vi "sensitivity mso Measurement.vi"(0 "OSC":refnum<visa-resource-name>, 2 "Sensor Threshold Setting":dbl=1.005, 5 "Pace Voltage":dbl=1.5 format="%#_13g", 7 "Waveform Generator":refnum<visa-resource-name>, 9 "Delay":u32=8000, 11 "error in (no error)":errorcluster, 12 "Pace interval":dbl) -> (6 "Raw Data with OSC":waveform(dbl)[](array[waveform]), 10 "CH1 Waveform":waveform(dbl)(graph), 14 "Sensor Threshold":dbl, 15 "CH3 Waveform":waveform(dbl)(graph))   [LabVIEW 2016]
uses:
  <instrlib>/Agilent 6000 Series/Agilent 6000 Series.lvlib
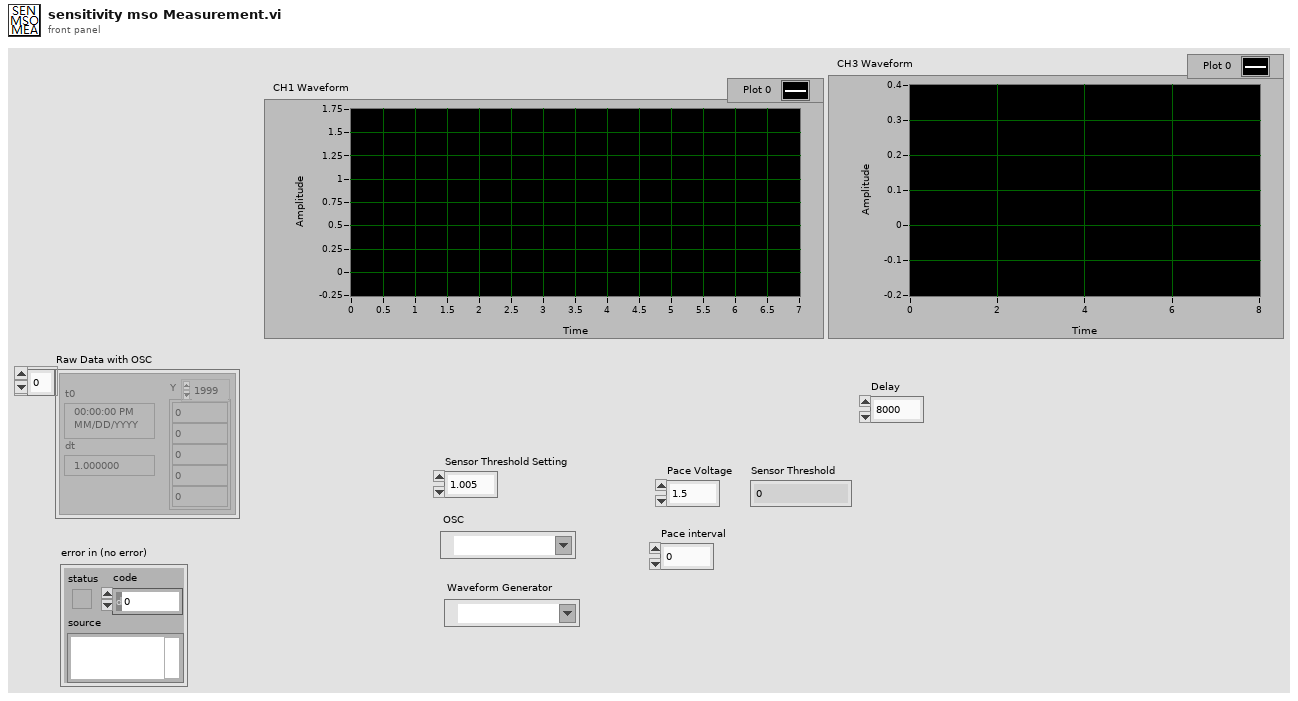
[diagram p1: front panel]
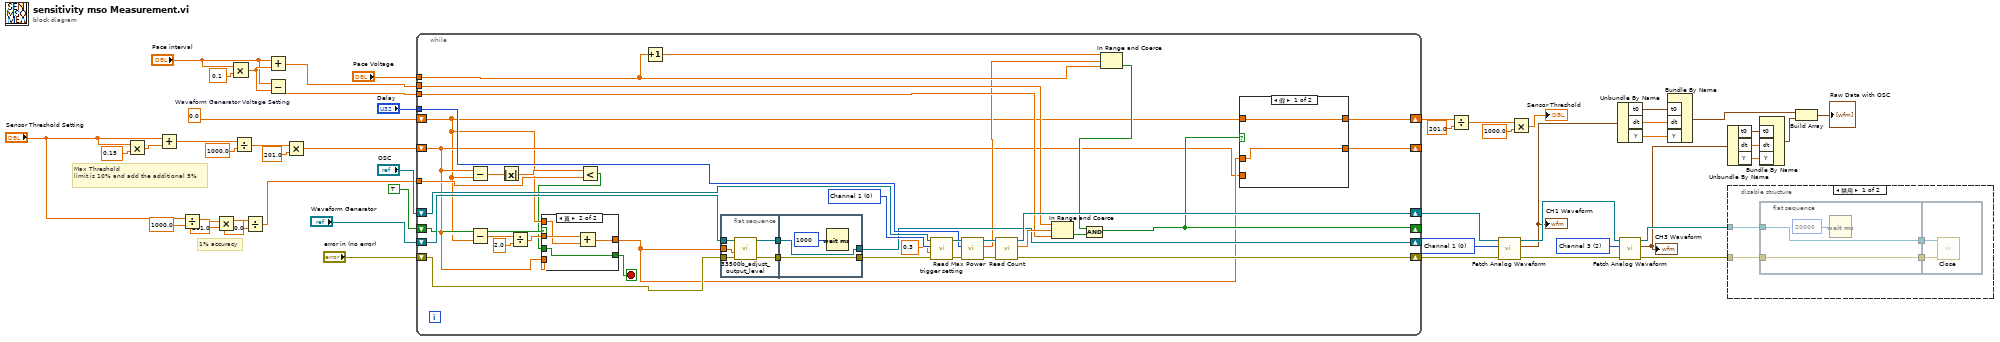
[diagram p0: block diagram]
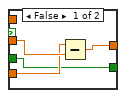
[diagram p2: hidden frame]
diagram:
  w9 = 0.0  # Waveform Generator Voltage Setting
  w48 = u16 2 items=["Channel 1", "Channel 2", "Channel 3", "Channel 4", "Math"] ("Source (0: Channel 1)")
  w50 = u16 0 items=["Channel 1", "Channel 2", "Channel 3", "Channel 4", "Math"] ("Source (0: Channel 1)")
  # "Max Threshold\nlimit is 10% and add the additional 5%"
  # "1% accuracy"
  n1 = Multiply(x="Sensor Threshold Setting", y=0.15) -> (x*y=w10:dbl)
  n2 = Add(x="Sensor Threshold Setting", y=w10) -> (x+y=w19:dbl)
  n3 = Divide(x="Sensor Threshold Setting", y=1000.0) -> (x/y=w5:dbl)
  n4 = Multiply(x=w5, y=201.0) -> (x*y=w3:dbl)
  n5 = Multiply(x="Pace interval", y=0.1) -> (x*y=w15:dbl)
  n6 = Divide(x=w19, y=1000.0) -> (x/y=w17:dbl)
  n7 = Divide(x=w3, y=100.0) -> (x/y=w1:dbl)
  n8 = Add(x="Pace interval", y=w15) -> (x+y=w13:dbl)
  n9 = Subtract(x="Pace interval", y=w15) -> (x-y=w14:dbl)
  n10 = Multiply(x=w17, y=201.0) -> (x*y=w23:dbl)
  n11 = while {
    shift-right: [w76] -> w31
    shift-left: "OSC" -> [w89]
    shift-right: [w77] -> w30
    shift-left: "error in (no error)" -> [w65]
    tunnel: "Delay" -> [w85]
    tunnel: "Pace Voltage" -> [w63]
    shift-right: [w59] -> w26
    shift-left: w9 -> [w53]
    shift-right: [w70] -> _
    shift-left: "Waveform Generator" -> [w71]
    shift-right: [w56] -> _
    shift-left: w23 -> [w54]
    tunnel: w14 -> [w73]
    tunnel: w13 -> [w72]
    shift-right: [w60] -> _
    shift-left: TRUE -> [w55]
    tunnel: w1 -> [w66]
    stop <- w51 stop-if-true
    w88 = u16 0 items=["Channel 1", "Channel 2", "Channel 3", "Channel 4", "DIG 0", "DIG 1", "DIG 2", "DIG 3", "DIG 4", "DIG 5", "DIG 6", "DIG 7", "DIG 8", "DIG 9", "DIG 10", "DIG 11", "DIG 12", "DIG 13", "DIG 14", "DIG 15", "Line", "External"] ("Trigger Source (0: Channel 1)")
    n12 = Subtract(x=w54, y=w53) -> (x-y=w81:dbl)
    n13 = Subtract(x=w54, y=w53) -> (x-y=w84:dbl)
    n14 = Absolute Value(x=w81) -> (abs(x)=w80:dbl)
    n15 = Divide(x=w84, y=2.0) -> (x/y=w58:dbl)
    n16 = Less?(x=w80, y=w66) -> (x < y?=w52:bool)
    n17 = case shown="真" w55 {
      tunnel: w58 -> [w92 w97]
      tunnel: [w93 w96] -> w57
      tunnel: w54 -> [w91 _]
      tunnel: w53 -> [_ w95]
      tunnel: w52 -> [w90 w94]
      tunnel: [w90 w94] -> w51
      frame False {
        n18 = Subtract(x=w91, y=w92) -> (x-y=w93:dbl)
      }
      frame True {
        n19 = Add(x=w97, y=w95) -> (x+y=w96:dbl)
      }
    }
    n20 = Increment(x=w63) -> (x+1=w64:dbl)
    n21 = flat-sequence {
      tunnel: w71 -> [w106]
      tunnel: w65 -> [w104]
      tunnel: [w105] -> w69
      tunnel: [w103] -> w68
      tunnel: w57 -> [w102]
      tunnel: [w109] -> w70
      tunnel: w69 -> [w109]
      tunnel: w68 -> [w107]
      tunnel: [w107] -> w67
      frame #0 {
        n22 = call "33500b_adjust_output_level.vi"("错误输入（无错误）"=w104, "Amp(vpp)"=w102, "Waveform Generator"=w106) -> ("错误输出"=w103:errorcluster, "Waveform Generator"=w105:refnum<visa-resource-name>)  [unwired: 7 in]
      }
      frame #1 {
        n23 = Wait (ms)(milliseconds to wait=u32 1000 ("等待时间（毫秒）")) -> ()  [unwired: 1 out]
      }
    }
    n24 = call "trigger setting.vi"("error in (no error)"=w67, "Trigger Level (0.0 V)"=0.3, "Trigger Source (0: Channel 1)"=w88, "OSC"=w89) -> ("error out"=w86:errorcluster, "OSC"=w87:refnum<visa-resource-name>)  [unwired: 6 in]
    n25 = call "Read Max Power.vi"("错误输入（无错误）"=w86, "Delay"=w85, "OSC Input"=w87) -> ("错误输出"=w78:errorcluster, "Pace Max Amp"=w62:dbl, "OSC Output"=w79:refnum<visa-resource-name>)  [unwired: 6 in]
    n26 = call "Read Count.vi"("错误输入（无错误）"=w78, "OSC Input"=w79) -> ("错误输出"=w77:errorcluster, "Pace Interval"=w75:dbl, "OSC Output"=w76:refnum<visa-resource-name>)  [unwired: 7 in]
    n27 = In Range and Coerce(upper limit=w72, x=w75, lower limit=w73) -> (In Range?=w74:bool)  [unwired: 1 out]
    n28 = In Range and Coerce(upper limit=w64, x=w62, lower limit=w63) -> (In Range?=w61:bool)  [unwired: 1 out]
    n29 = Compound Arithmetic op=AND ("复合运算")(w61, w74) -> (w60:bool)
    n30 = case shown="假" w60 {
      tunnel: w57 -> [w99 w101]
      tunnel: [w98 w101] -> w59
      tunnel: w54 -> [_ w100]
      tunnel: [w99 w100] -> w56
      tunnel: w53 -> [w98 _]
      frame False {
      }
      frame True {
      }
    }
  }
  n31 = Divide(x=w26, y=201.0) -> (x/y=w22:dbl)
  n32 = call <instrlib>:"Fetch Analog Waveform.vi"("error in (no error)"=w30, "Source (0: Channel 1)"=w50, "VISA resource name"=w31) -> ("error out"=w45:errorcluster, "Waveform Data"=w44:waveform(dbl), "VISA resource name out"=w49:refnum<visa-resource-name>)  [unwired: 6 in]
  "CH1 Waveform" <- w44
  n33 = Multiply(x=w22, y=1000.0) -> (x*y=→"Sensor Threshold":dbl)
  n34 = Unbundle By Name(w44) -> ("t0"=w43:timestamp, "dt"=w42:dbl, "Y"=w41:dbl[])
  n35 = call <instrlib>:"Fetch Analog Waveform.vi"("error in (no error)"=w45, "Source (0: Channel 1)"=w48, "VISA resource name"=w49) -> ("error out"=w46:errorcluster, "Waveform Data"=w37:waveform(dbl), "VISA resource name out"=w47:refnum<visa-resource-name>)  [unwired: 6 in]
  "CH3 Waveform" <- w37
  n36 = Bundle By Name("t0"=w43, "dt"=w42, "Y"=w41) -> (w36:waveform(dbl))  [unwired: 1 in]
  n37 = Unbundle By Name(w37) -> ("t0"=w38:timestamp, "dt"=w39:dbl, "Y"=w40:dbl[])
  n38 = disable-structure shown="禁用" {
    disable-tunnel: w47 -> [w111 _]
    disable-tunnel: w46 -> [w110 _]
    frame Disabled {
      n39 = flat-sequence {
        tunnel: w110 -> [w115]
        tunnel: w111 -> [w116]
        tunnel: [w116] -> w113
        tunnel: [w115] -> w112
        tunnel: w113 -> [w118]
        tunnel: w112 -> [w117]
        frame #0 {
          n40 = Wait (ms)(milliseconds to wait=u32 20000 ("等待时间（毫秒）")) -> ()  [unwired: 1 out]
        }
        frame #1 {
          n41 = call <instrlib>:"Close.vi"("error in (no error)"=w117, "VISA resource name"=w118) -> ()  [unwired: 9 in, 1 out]
        }
      }
    }
    frame Enabled {
    }
  }
  n42 = Bundle By Name("t0"=w38, "dt"=w39, "Y"=w40) -> (w35:waveform(dbl))  [unwired: 1 in]
  n43 = Build Array(w36, w35) -> (→"Raw Data with OSC":waveform(dbl)[])
